vi "Mock VS engine.vi"() -> ()   [LabVIEW 2014]
uses:
  Shared/UEGO Sim Shared.lvlib
  UEGO Sim Engine.lvlib
  <vilib>/NI Veristand/Custom Device API/Custom Device Item Ref.ctl
  <vilib>/NI Veristand/Custom Device API/Custom Device API.lvlib
  Shared/VS output channels.ctl
  <instrlib>/ni272xReferenceVIs/ni272xReferenceVIs.llb/ni272x Write Resistance 1Chan 1Samp.vi
  <instrlib>/ni272xReferenceVIs/ni272xReferenceVIs.llb/ni272x Connector Identifier.ctl
  <instrlib>/ni272xReferenceVIs/ni272xReferenceVIs.llb/ni272x Connect to Connector 1Chan.vi
  <vilib>/rvi/interface/nirviOpenFPGA/nirviOpenFPGA.xnode
  FPGA Bitfiles/UEGOSimCustomDev_FPGATarget_examplefpgacode_CnYhSZw3IHk.lvbitx
  FPGA/example fpga code.vi
  <vilib>/FPGAPlugInAG/PXI-7854R/niLvFpga_Open_PXI-7854R.vi
  <vilib>/rvi/interface/common/dynamic/niFpgaDynamicAddResources.vi
  <vilib>/rvi/interface/nirviMethod/nirviMethod.xnode
  <vilib>/FPGAPlugInAG/Dynamic/niLvFpga_Reset_Dynamic.vi
  <vilib>/rvi/interface/nirviCloseFPGA/nirviCloseFPGA.xnode
  <vilib>/FPGAPlugInAG/Dynamic/niLvFpga_Close_Dynamic.vi
  Shared/VS input channels.ctl
panel:
  out "coerced resistance (ohms)":dbl
  in  "DAQmx Device Name":tag="PXI1Slot8"
  in  "CD Inputs":T1[](array[typedef])=[{"lambda"=1.0, "thermal reset"=0.0, "PWM timeout"=50000.0, "PWM threshold"=200.0, "Heater Invert"=0.0}, {"lambda"=1.0, "thermal reset"=0.0, "PWM timeout"=0.0, "PWM threshold"=0.0, "Heater Invert"=0.0}, {"lambda"=1.0, "thermal reset"=0.0, "PWM timeout"=0.0, "PWM threshold"=0.0, "Heater Invert"=0.0}, {"lambda"=1.0, "thermal reset"=0.0, "PWM timeout"=0.0, "PWM threshold"=0.0, "Heater Invert"=0.0}]
  out "CD Ouputs":T2[](array[typedef])
  in  "Stop Button":bool
  in  "thermal model rate":dbl=50.0 format="%#_13g"
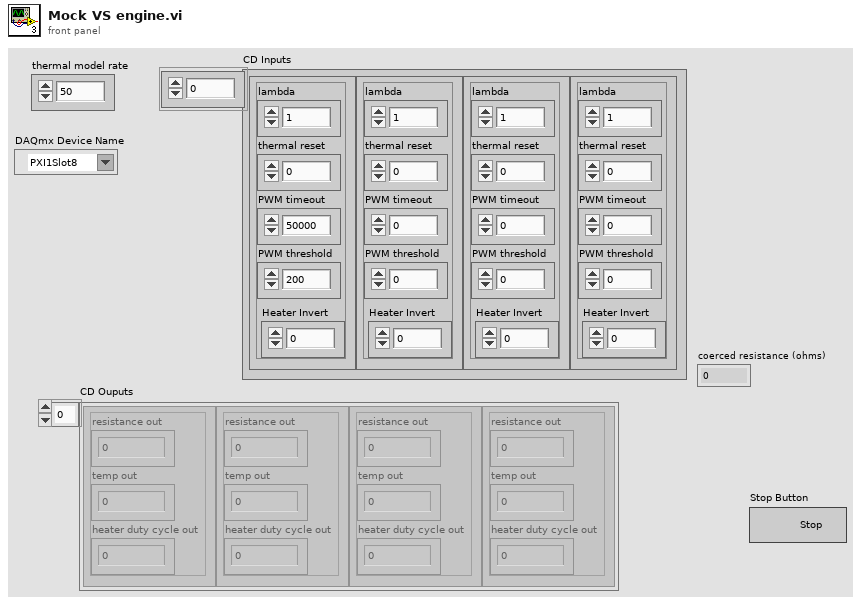
[diagram p1: front panel]
types:
  T1 = typedef "UEGO Sim Shared.lvlib/VS input channels.ctl" = cluster{"lambda":dbl, "thermal reset":dbl, "PWM timeout":dbl, "PWM threshold":dbl, "Heater Invert":dbl}
  T2 = typedef "UEGO Sim Shared.lvlib/VS output channels.ctl" = cluster{"resistance out":dbl, "temp out":dbl, "heater duty cycle out":dbl}
  T3 = typedef "Custom Device API.lvlib/Custom Device Item Ref.ctl" = u64
  T4 = cluster{"read mode":enum16{"polling", "blocking"}, "write mode":enum16{"polling", "blocking"}}
  T5 = typedef "UEGO Sim Shared.lvlib/sensor models" = enum16{"Narrow Band", "Bosch 4.2", "Bosch 4.9"}
  T6 = typedef "ni272x Reference.ctl" = refnum<k20>
  T7 = typedef "ni272x Connector Identifier.ctl" = enum8{"DUT Connector", "DMM Test Connector"}
  T8 = cluster{"ambient T, sensor t0, and heat params[0]":dbl, "ambient T, sensor t0, and heat params[1]":dbl, "ambient T, sensor t0, and heat params[2]":dbl}
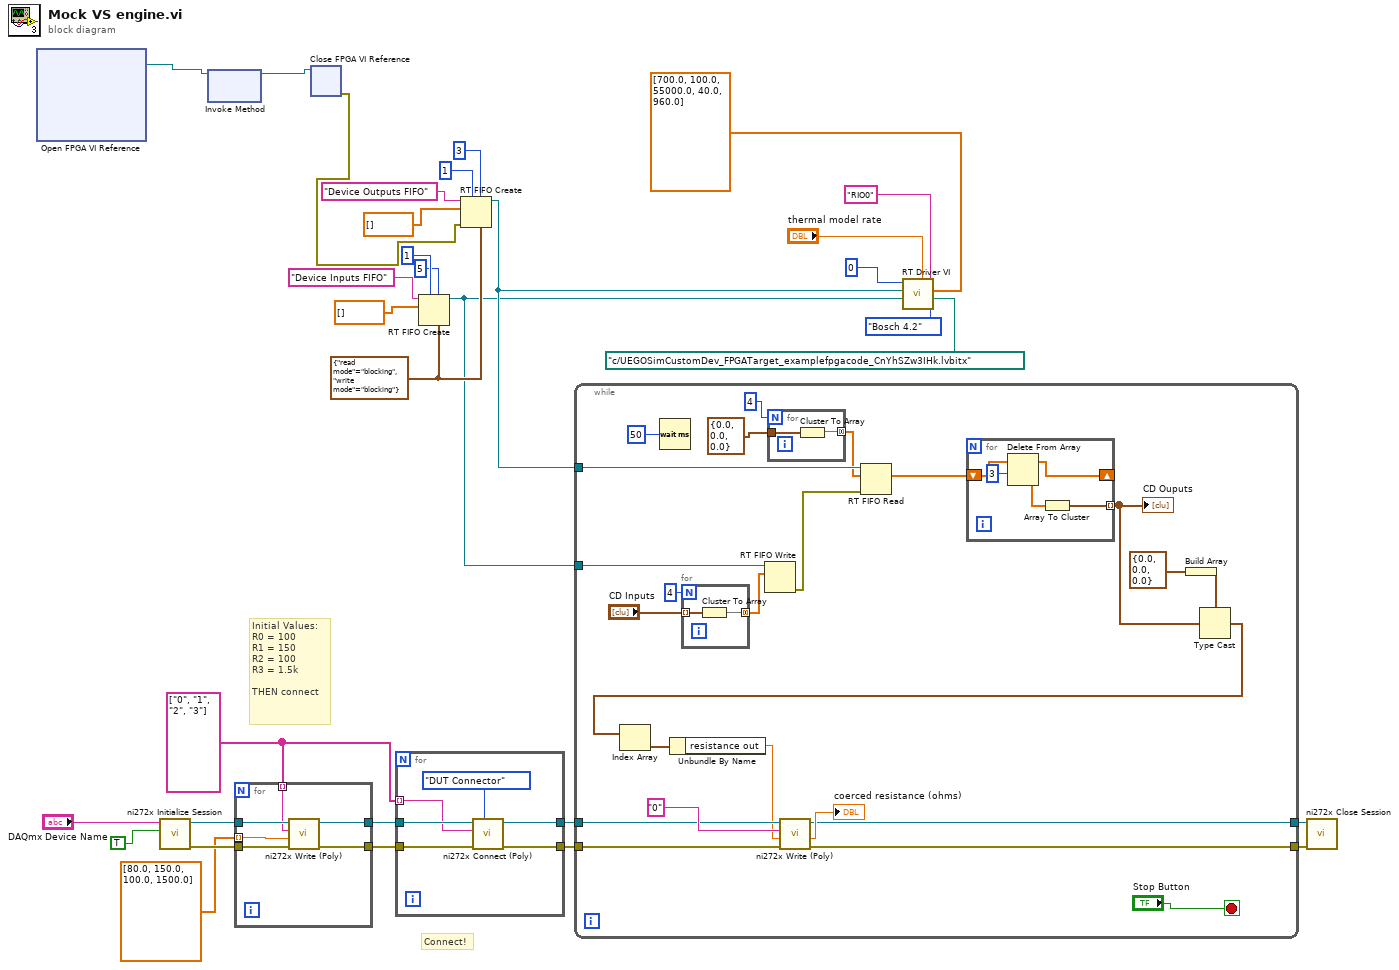
[diagram p0: block diagram]
diagram:
  w8 = string[] ["0", "1", "2", "3"]
  w30 = T4 {"read mode"=enum."blocking", "write mode"=enum."blocking"} ("r/w modes (polling,polling)")
  # "Connect!"
  # "Initial Values:\nR0 = 100\nR1 = 150\nR2 = 100\nR3 = 1.5k\n\nTHEN connect"
  n1 = xnode "Open FPGA VI Reference"() -> ("FPGA VI Reference Out"=w3:refnum<k20>)  [unwired: 2 in, 1 out]
  n2 = call <instrlib>:"ni272x Initialize Session.vi"("reset device (T)"=TRUE, "DAQmx Device Name"="DAQmx Device Name") -> ("error out"=w10:errorcluster, "instrument handle out"=w13:T6)  [unwired: 8 in]
  n3 = xnode "Invoke Method"("FPGA VI Reference In"=w3) -> ("FPGA VI Reference Out"=w2:refnum<k20>)  [unwired: 1 in, 1 out]
  n4 = for {
    tunnel: w13 -> [w38]
    tunnel: [w37] -> w12
    tunnel: [w36] -> w11
    tunnel: w10 -> [w35]
    tunnel: w8 -> [w34] mode=indexing
    tunnel: dbl[] [80.0, 150.0, 100.0, 1500.0] -> [w33] mode=indexing
    n5 = call-poly <instrlib>:"ni272x Write (Poly).vi"("error in (no error)"=w35, "requested resistance (ohms)"=w33, "resistor channel"=w34, "instrument handle"=w38) -> ("error out"=w36:errorcluster, "instrument handle out"=w37:T6)  [unwired: 5 in, 1 out]
  }
  n6 = xnode "Close FPGA VI Reference"("FPGA VI Reference In"=w2) -> ("error out"=w1:errorcluster)  [unwired: 1 in]
  n7 = for {
    tunnel: [w44] -> w6
    tunnel: [w43] -> w7
    tunnel: w12 -> [w41]
    tunnel: w11 -> [w40]
    tunnel: w8 -> [w39] mode=indexing
    n8 = call-poly <instrlib>:"ni272x Connect (Poly).vi"("connector identifier"=ni272x_Connector_Identifier."DUT Connector", "error in (no error)"=w40, "resistor channel"=w39, "instrument handle"=w41) -> ("error out"=w44:errorcluster, "instrument handle out"=w43:T6)  [unwired: 6 in]
  }
  n9 = RT FIFO Create(0:"Device Inputs FIFO" ("Control Name"), 1:dbl[] [] ("ambient T, sensor t0, and heat params"), 4:u32 1 ("size (10)"), 6:u32 5 ("elements in array (1)"), 7:w30) -> (8:w21:refnum<k33>)  [unwired: 3 in, 2 out]
  n10 = RT FIFO Create(0:"Device Outputs FIFO" ("Control Name"), 1:dbl[] [] ("ambient T, sensor t0, and heat params"), 3:w1, 4:u32 1 ("size (10)"), 6:u32 3 ("elements in array (1)"), 7:w30) -> (8:w22:refnum<k33>)  [unwired: 2 in, 2 out]
  n11 = while {
    tunnel: w22 -> [w67]
    tunnel: w21 -> [w66]
    tunnel: w7 -> [w59]
    tunnel: w6 -> [w58]
    tunnel: [w57] -> w5
    tunnel: [w56] -> w4
    stop <- "Stop Button" stop-if-true
    n12 = Wait (ms)(milliseconds to wait=u32 50) -> ()  [unwired: 1 out]
    n13 = for {
      N: 4 -> [_]
      tunnel: "CD Inputs" -> [w77] mode=indexing
      tunnel: [w76] -> w54 mode=concatenating
      n14 = Cluster To Array(cluster=w77) -> (array=w76:dbl[])
    }
    n15 = RT FIFO Write(0:w66, 1:w54) -> (11:w62:errorcluster)  [unwired: 3 in, 3 out]
    n16 = for {
      N: 4 -> [_]
      tunnel: [w75] -> w65 mode=concatenating
      tunnel: T2 {"resistance out"=0.0, "temp out"=0.0, "heater duty cycle out"=0.0} ("VS output channels") -> [w74]
      n17 = Cluster To Array(cluster=w74) -> (array=w75:dbl[])
    }
    n18 = RT FIFO Read(0:w67, 1:w65, 3:w62) -> (9:w51:dbl[])  [unwired: 1 in, 4 out]
    n19 = for {
      shift-right: [w72] -> _
      shift-left: w51 -> [w73]
      tunnel: [w69] -> w50 mode=indexing
      n20 = Delete From Array(array=w73, length=3) -> (deleted portion=w70:dbl[], array with subset deleted=w72:dbl[])  [unwired: 1 in]
      n21 = Array To Cluster(array=w70) -> (cluster=w69:T8)
    }
    "CD Ouputs" <- w50
    n22 = Build Array(T2 {"resistance out"=0.0, "temp out"=0.0, "heater duty cycle out"=0.0} ("VS output channels")) -> (w47:T2[])
    n23 = Type Cast(type=w47, x=w50) -> (*(type *) &x=w48:T2[])
    n24 = Index Array(array=w48) -> (element=w46:T2)  [unwired: 1 in]
    n25 = Unbundle By Name(w46) -> ("resistance out"=w45:dbl)
    n26 = call-poly <instrlib>:"ni272x Write (Poly).vi"("error in (no error)"=w58, "requested resistance (ohms)"=w45, "resistor channel"="0", "instrument handle"=w59) -> ("error out"=w56:errorcluster, "coerced resistance (ohms)"=→"coerced resistance (ohms)":dbl, "instrument handle out"=w57:T6)  [unwired: 5 in]
  }
  n27 = call "RT Driver VI.vi"("Sensor Model"=sensor_models."Bosch 4.2", "bitfile address"=path "c:/UEGOSimCustomDev_FPGATarget_examplefpgacode_CnYhSZw3IHk.lvbitx", "ambient T, sensor t0, and heat params"=dbl[] [700.0, 100.0, 55000.0, 40.0, 960.0], "RIO address"="RIO0" ("Control Name"), "thermal model rate"="thermal model rate", "Device Inputs FIFO"=w21, "Device Outputs FIFO"=w22, "Device Reference"=T3 0) -> ()  [unwired: 4 in]
  n28 = call <instrlib>:"ni272x Close Session.vi"("error in (no error)"=w4, "instrument handle"=w5) -> ()  [unwired: 9 in, 1 out]
